vi "Teardown.vi"(8 "error in (no error)":errorcluster, 11 "LUnit Indexing Test Finder Test In":refnum<class "Indexing Test Finder Test.lvclass">) -> (0 "error out":errorcluster, 3 "LUnit Indexing Test Finder Test Out":refnum<class "Indexing Test Finder Test.lvclass">)   [LabVIEW 2020, in "LUnit Tests.lvlib" / "Indexing Test Finder Test.lvclass"]
uses:
  Indexing Test Finder Test.lvclass
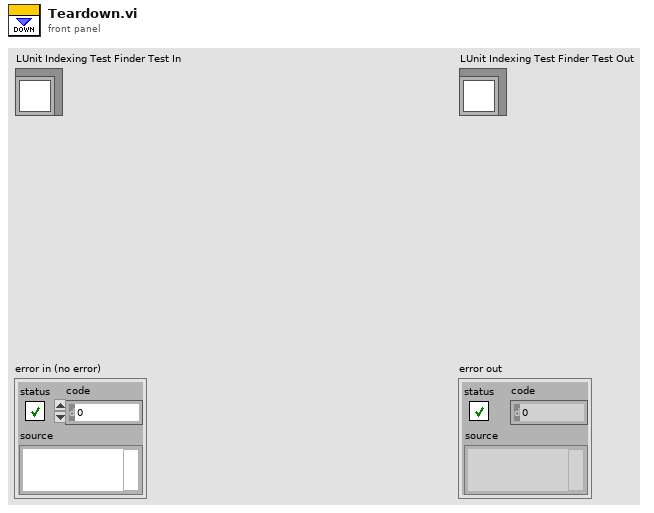
[diagram p1: front panel]
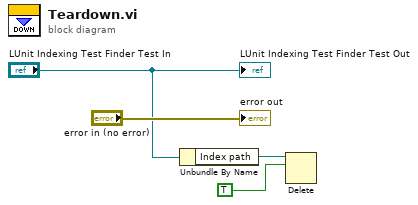
[diagram p0: block diagram]
diagram:
  n1 = Unbundle By Name("LUnit Indexing Test Finder Test In") -> ("Index path"=w2:path)
  n2 = Delete(path (use dialog)=w2, entire hierarchy (F)=TRUE) -> ()  [unwired: 3 in, 3 out]
  "error out" <- "error in (no error)"
  "LUnit Indexing Test Finder Test Out" <- "LUnit Indexing Test Finder Test In"
